vi "SystemController.API_TEMPLATE.vi"(8 "error in (no error)":errorcluster, 10 "myData":string, 11 "SystemController":refnum<class "SystemController.lvclass">) -> (0 "error out":errorcluster, 2 "Data out":string, 3 "SystemController out":refnum<class "SystemController.lvclass">)   [LabVIEW 2017]
doc: "---------------------------------------------------------------\nJKI State Machine Objects™\nhttp://jki.net/state-machine-objects/\nCopyright (C) 2005-2015, JKI <info@jki.net>\nALL RIGHTS RESERVEDJKI State Machine Objects (SMO) 1.0.0.5\nJKI - JKI\nCopyright (c) 2016, JKI"
uses:
  SystemController.lvclass
  C:/Program Files (x86)/National Instruments/LabVIEW 2017/vi.lib/JKI/JKI SMO/SMO/SMO.lvclass
panel:
  # "For instructions on how to use the JKI State Machine Objects, examples and video tutorials, visit:\nhttp://jki.net/state-machine-objects/\n\nJKI State Machine Objects™\nhttp://jki.net/state-machine-objects/\nCopyright (C) 2005-2015, JKI <info@jki.net>\nALL RIGHTS RESERVED"
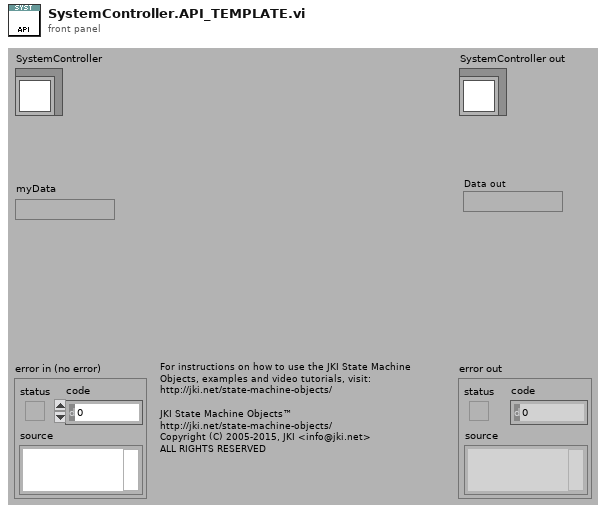
[diagram p1: front panel]
types:
  T1 = typedef "SystemController.lvclass/PrivateData--Ref.ctl" = refnum<data-value>
  T2 = typedef "SystemController.lvclass/PrivateData--Cluster.ctl" = cluster{"Configuration":T3, "Dependencies":T7, "Public Events":T8, "Processed Image Buffer":T9[]}
  T3 = typedef "SystemController.lvclass/Configuration--Cluster.ctl" = cluster{"Camera":T4, "Find Eyes":bool, "Acquisition Rate (ms)":i32, "Image Buffer Length":i32}
  T4 = typedef "SystemController.lvclass/CameraConfig--Cluster.ctl" = cluster{"Simulate Camera":bool, "IMAQ Camera":T5, "Simulated Image Folder":path}
  T5 = typedef "Camera_IMAQdx.lvclass/Configuration--Cluster.ctl" = cluster{"Camera Interface Name":string, "Number of Buffers":u32, "Image Name":string, "Image Type":T6}
  T6 = typedef "Image Type" = u32
  T7 = typedef "SystemController.lvclass/Dependencies--Cluster.ctl" = cluster{"Camera":refnum<class "Camera.lvclass">, "ImageFacialDetection":refnum<class "ImageFacialDetection.lvclass">}
  T8 = typedef "SystemController.lvclass/PublicEvents--Cluster.ctl" = cluster{"UIClosed":refnum<user-event>}
  T9 = typedef "IMAQ Image.ctl" = refnum<image>
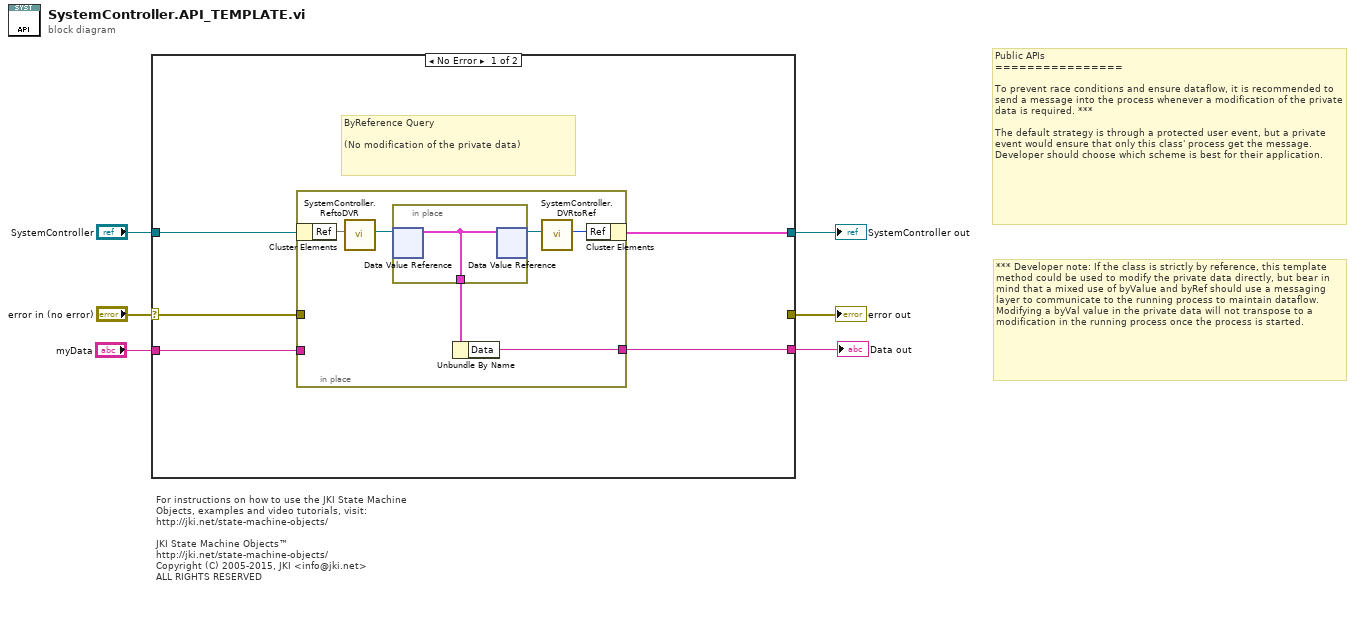
[diagram p0: block diagram]
diagram:
  # "*** Developer note: If the class is strictly by reference, this template method could be used to modify the private data directly, but bear in mind that a mixed use of byValue and byRef should use a messaging layer to communicate to the running process to maintain dataflow. Modifying a byVal value in the private data will not transpose to a modification in the running process once the process is started."
  # "Public APIs\n================\n\nTo prevent race conditions and ensure dataflow, it is recommended to send a message into the process whenever a modification of the private data is required. ***\n\nThe default strategy is through a protected user event, but a private event would ensure that only this class' process get the message. Developer should choose which scheme is best for their application."
  # "For instructions on how to use the JKI State Machine Objects, examples and video tutorials, visit:\nhttp://jki.net/state-machine-objects/\n\nJKI State Machine Objects™\nhttp://jki.net/state-machine-objects/\nCopyright (C) 2005-2015, JKI <info@jki.net>\nALL RIGHTS RESERVED"
  n1 = case shown="No Error" "error in (no error)" {
    selector: "error in (no error)" -> [w10 w19]
    tunnel: "SystemController" -> [w8 w20]
    tunnel: [_ w19] -> w5
    tunnel: [w9 w20] -> w4
    tunnel: "myData" -> [w11 _]
    tunnel: [w7 _] -> w1
    frame No Error {
      # "ByReference Query\n\n(No modification of the private data)"
      n2 = in-place {
        in-place-border: w10 -> [_]
        in-place-border: w11 -> [_]
        in-place-border: [w12] -> w7
        n3 = in-place-cluster #1(w8) -> ("Ref"=w16)
        n4 = call "SystemController.ReftoDVR.vi"("Ref"=w16) -> ("Ref"=w17:T1)  [unwired: 10 in]
        n5 = in-place {
          in-place-border: [w18] -> w13
          n6 = in-place-dvr #2(w17) -> (w18:T2)  [unwired: 1 out]
          n7 = in-place-dvr #2(w18) -> (w15:T1)  [unwired: 1 out]
        }
        n8 = Unbundle By Name(w13) -> ("Data"=w12:string)
        n9 = call "SystemController.DVRtoRef.vi"("Ref"=w15) -> ("Ref"=w14:u32)  [unwired: 10 in]
        n10 = in-place-cluster #1("Ref"=w14) -> (w9:cluster{})
      }
    }
    frame Error {
    }
  }
  "error out" <- w5
  "SystemController out" <- w4
  "Data out" <- w1
